vi "Obtain.vi"(8 "error in (no error)":errorcluster, 11 "ID in":i32) -> (0 "error out":errorcluster, 2 "Self":T1, 3 "Instance":T2)   [LabVIEW 2022 SP3, in "Shared.lvlib"]
uses:
  Shared.lvlib
  Controls/Instance.ctl
  Controls/Global.ctl
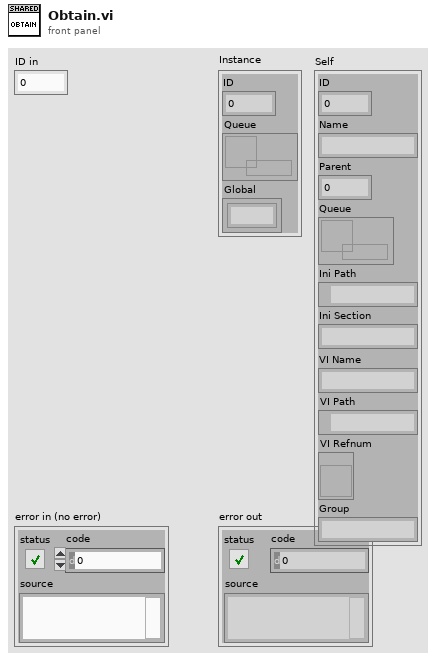
[diagram p1: front panel]
types:
  T1 = typedef "Shared.lvlib/Global.ctl" = cluster{"ID":i32, "Name":string, "Parent":i32, "Queue":refnum<queue>, "Ini Path":path, "Ini Section":string, "VI Name":string, "VI Path":path, "VI Refnum":refnum<vi>, "Group":string}
  T2 = typedef "Shared.lvlib/Instance.ctl" = cluster{"ID":i32, "Queue":refnum<queue>, "Global":refnum<k1>}
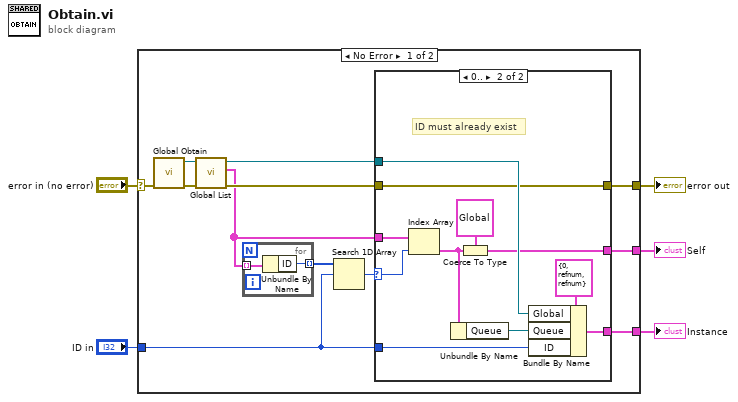
[diagram p0: block diagram]
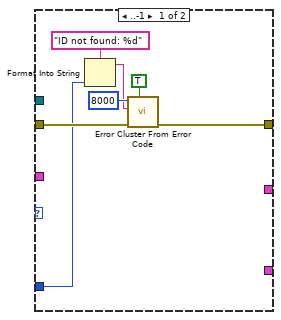
[diagram p2: hidden frame]
diagram:
  n1 = case shown="No Error" "error in (no error)" {
    selector: "error in (no error)" -> [w11 w38]
    tunnel: [w15 _] -> w4
    tunnel: "ID in" -> [w14 _]
    tunnel: [w13 w38] -> w2
    tunnel: [w12 _] -> w1
    frame No Error {
      n2 = call "Global Obtain.vi"("error in (no error)"=w11) -> ("error out"=w9:errorcluster, "Global"=w10:refnum<k1>)  [unwired: 8 in, 1 out]
      n3 = call "Global List.vi"("error in (no error)"=w9, "Global in"=w10) -> ("error out"=w7:errorcluster, "Instances"=w6:T1[], "Global out"=w8:refnum<k1>)  [unwired: 7 in]
      n4 = for {
        tunnel: w6 -> [w37] mode=indexing
        tunnel: [w36] -> w17 mode=indexing
        n5 = Unbundle By Name(w37) -> ("ID"=w36:i32)
      }
      n6 = Search 1D Array(1D array=w17, element=w14) -> (index of element=w16:i32)  [unwired: 1 in]
      n7 = case shown="0.." w16 {
        selector: w16 -> [_ w34]
        tunnel: w6 -> [_ w35]
        tunnel: [_ w31] -> w15
        tunnel: w8 -> [_ w30]
        tunnel: w7 -> [w24 w29]
        tunnel: w14 -> [w20 w32]
        tunnel: [w23 w29] -> w13
        tunnel: [_ w25] -> w12
        frame ..-1 {
          n8 = Format Into String(format string="ID not found: %d", w20) -> (resulting string=w18:string)  [unwired: 2 in, 1 out]
          n9 = call <vilib>:"Error Cluster From Error Code.vi"("show call chain? (False)"=TRUE, "error in (no error)"=w24, "error message (\"\")"=w18, "error code (0)"=8000) -> ("error out"=w23:errorcluster)  [unwired: 5 in]
        }
        frame 0.. {
          # "ID must already exist"
          n10 = Index Array(array=w35, index=w34) -> (element=w26:T1)
          n11 = Unbundle By Name(w26) -> ("Queue"=w28:refnum<queue>)
          n12 = Coerce To Type(0:w26, 1:T1 {"ID"=0, "Name"="", "Parent"=0, "Queue"=refnum, "Ini Path"=path "", "Ini Section"="", "VI Name"="", "VI Path"=path "", "VI Refnum"=refnum, "Group"=""} ("Global")) -> (2:w25:T1)
          n13 = Bundle By Name(cluster=T2 {"ID"=0, "Queue"=refnum, "Global"=refnum} ("Instance"), "Global"=w30, "Queue"=w28, "ID"=w32) -> (w31:T2)
        }
      }
    }
    frame Error {
    }
  }
  "error out" <- w2
  "Instance" <- w4
  "Self" <- w1
